vi "Decorator.vi"(8 "error in (no error)":errorcluster, 10 "DecoratorData in":refnum<class "Data.lvclass">, 11 "DataVer3 in":refnum<class "DataVer3.lvclass">) -> (0 "error out":errorcluster, 3 "DataVer3 out":refnum<class "DataVer3.lvclass">)   [LabVIEW 2013, in "DataVer3.lvclass"]
uses:
  DataVer3.lvclass
  Data.lvclass/Data.lvclass
  DataVer3.lvclass/DataVer3.ctl
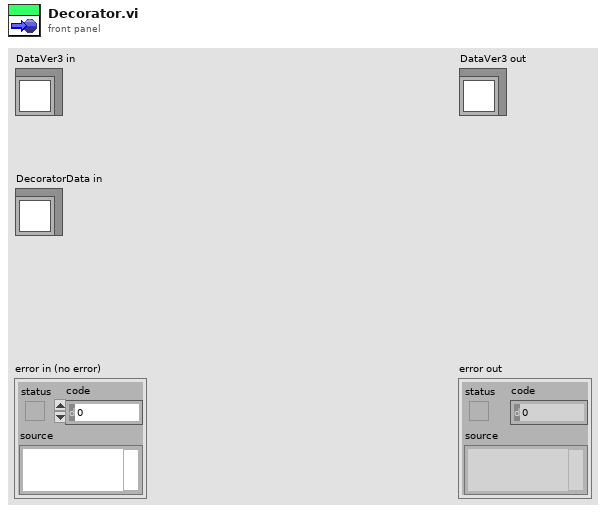
[diagram p1: front panel]
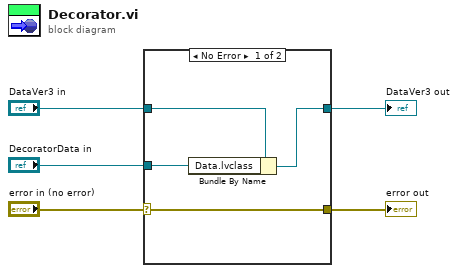
[diagram p0: block diagram]
diagram:
  n1 = case shown="No Error" "error in (no error)" {
    selector: "error in (no error)" -> [w9 w11]
    tunnel: [w9 w11] -> w1
    tunnel: [w6 w10] -> w2
    tunnel: "DataVer3 in" -> [w7 w10]
    tunnel: "DecoratorData in" -> [w8 _]
    frame No Error {
      n2 = Bundle By Name(cluster=w7, "Data.lvclass"=w8) -> (w6:refnum<class "DataVer3.lvclass">)
    }
    frame Error {
    }
  }
  "error out" <- w1
  "DataVer3 out" <- w2
